vi "VGI Init GPIO.vi"(7 "PinMode":u32, 9 "PinMask":u16, 10 "DevIndex":i32, 11 "DevType":i32) -> (3 "function return":i32)   [LabVIEW 2010, in "ControlGPIO.lvlib"]
doc: "int WINAPI VGI_InitGPIO(int DevType, int DevIndex, unsigned short PinMask, unsigned int PinMode);"
uses:
  ControlGPIO.lvlib
  ControlGPIO/Ginkgo_Driver.dll
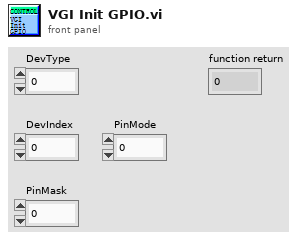
[diagram p1: front panel]
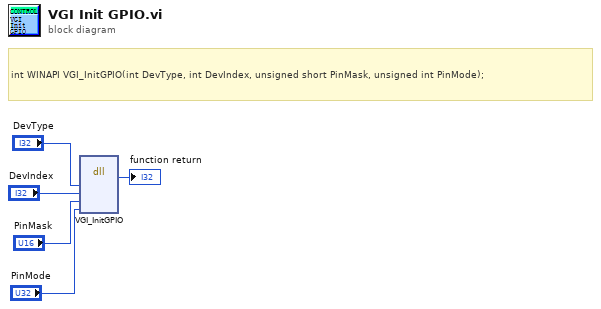
[diagram p0: block diagram]
diagram:
  # "int WINAPI VGI_InitGPIO(int DevType, int DevIndex, unsigned short PinMask, unsigned int PinMode);"
  n1 = dll-call lib="E:/Project/vt_ginkgo/truck/Ginkgo Driver/vs2010/Ginkgo_USB-I2C&SPI&CAN_API_v2.0.3.3/lib/labview_32bit/ControlGPIO/Ginkgo_Driver.*" fn="VGI_InitGPIO"("DevType"="DevType", "DevIndex"="DevIndex", "PinMask"="PinMask", "PinMode"="PinMode") -> (→"function return":i32)  [unwired: 7 in, 2 out]
